vi "UPdate Mask Paramter.vi"(8 "Color Box":u32(colorbox), 9 "Enabled/Disabled":bool, 10 "ROIName":string[](array[string]), 11 "Cluster in":refnum<vi>) -> (3 "Cluster out":refnum<vi>)   [LabVIEW 2019]
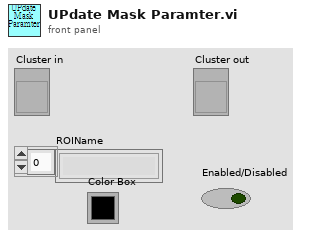
[diagram p1: front panel]
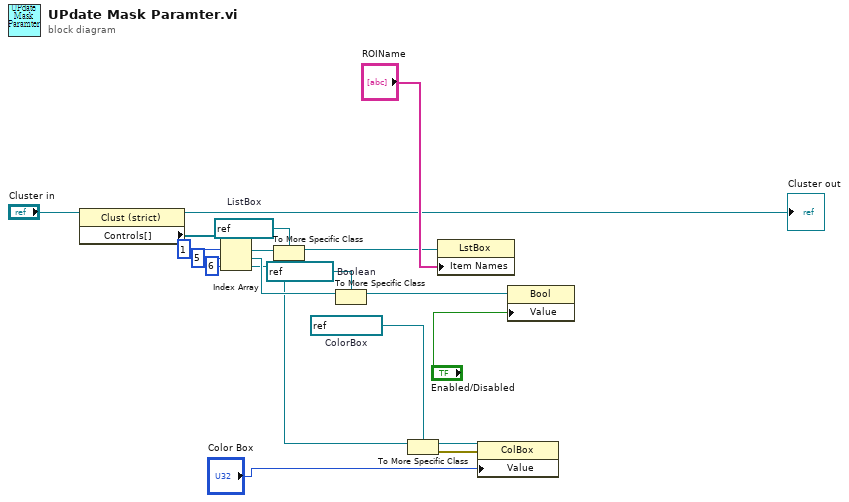
[diagram p0: block diagram]
diagram:
  w4 = refnum<vi> refnum  # ColorBox
  w9 = refnum<vi> refnum  # Boolean
  w13 = refnum<vi> refnum  # ListBox
  n1 = property class="Clust (strict)"(reference="Cluster in") -> (reference out=→"Cluster out":refnum<vi>, "Controls[]"=w10:refnum<vi>[])  [unwired: 1 in, 1 out]
  n2 = Index Array(array=w10, index #1=1 ("index"), index #2=5 ("index"), index #3=6 ("index")) -> (element #1=w12:refnum<vi>, element #2=w8:refnum<vi>, element #3=w5:refnum<vi>)
  n3 = To More Specific Class(target class=w13, reference=w12) -> (specific class reference=w14:refnum<vi>)  [unwired: 1 in, 1 out]
  n4 = To More Specific Class(target class=w9, reference=w8) -> (specific class reference=w7:refnum<vi>)  [unwired: 1 in, 1 out]
  n5 = To More Specific Class(target class=w4, reference=w5) -> (specific class reference=w3:refnum<vi>, error out=w2:errorcluster)  [unwired: 1 in]
  n6 = property class="LstBox"(reference=w14, "Item Names"="ROIName") -> ()  [unwired: 1 in, 2 out]
  n7 = property class="ColBox"(reference=w3, error in=w2, "Value"="Color Box") -> ()  [unwired: 2 out]
  n8 = property class="Bool"(reference=w7, "Value"="Enabled/Disabled") -> ()  [unwired: 1 in, 2 out]
